vi "Transmitter_type.vi"(8 "error in (no error)":errorcluster, 10 "Transmitter":string="001", 11 "VISA resource name":refnum<visa-resource-name>) -> (0 "error out":errorcluster, 1 "Vacuum gauge type":string, 2 "Transmitter type":string, 3 "VISA resource name 2":refnum<visa-resource-name>)   [LabVIEW 2010]
panel:
  out "concatenated string":string
  out "octal integer string":string
  out "sum":u8
  out "unsigned byte array":u8[](array[numeric])
  out "*(type *) &x":string
  out "Numeric":u8
  out "read buffer":string
  out "return count":u32
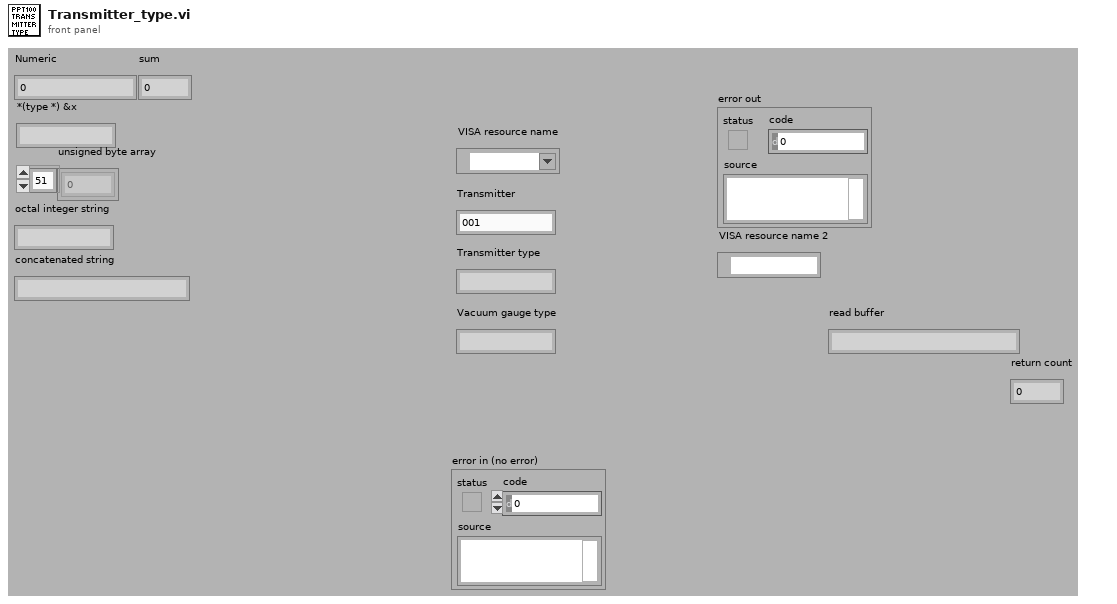
[diagram p1: front panel]
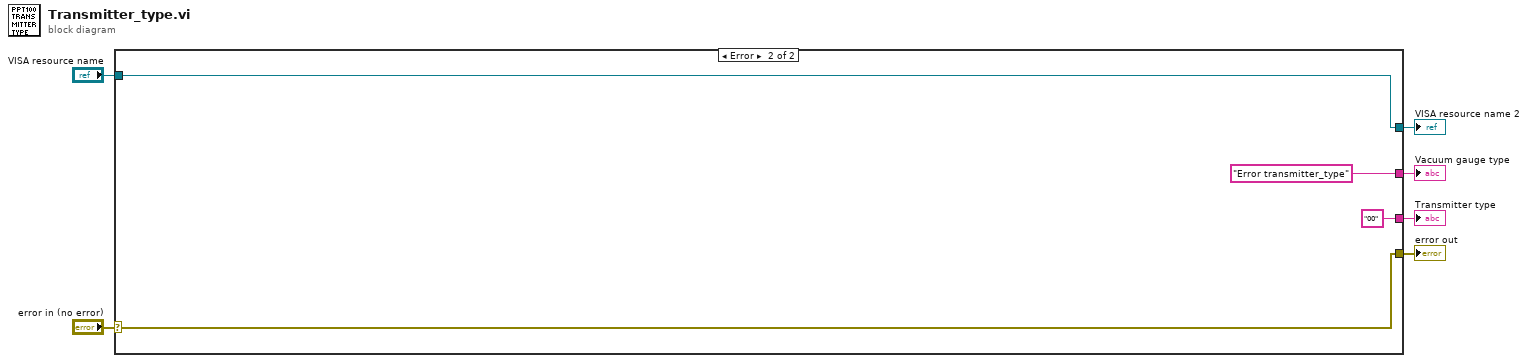
[diagram p0: block diagram]
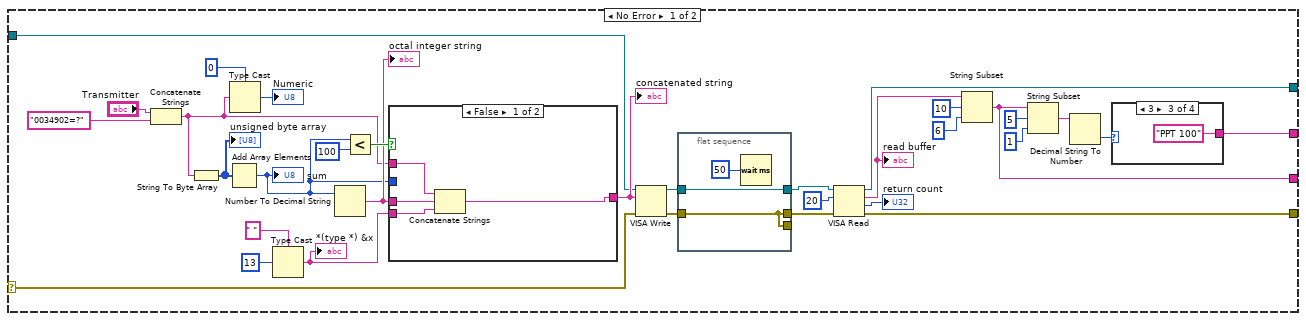
[diagram p2: hidden frame]
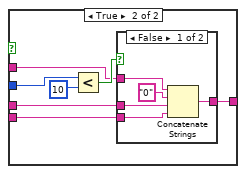
[diagram p3: hidden frame]
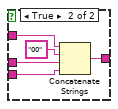
[diagram p4: hidden frame]
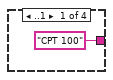
[diagram p5: hidden frame]
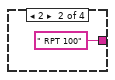
[diagram p6: hidden frame]
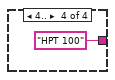
[diagram p7: hidden frame]
diagram:
  n1 = case shown="Error" "error in (no error)" {
    selector: "error in (no error)" -> [w10 w70]
    tunnel: "VISA resource name" -> [w11 w71]
    tunnel: [w37 w70] -> w5
    tunnel: [w36 w71] -> w3
    tunnel: [w28 "00" ("read buffer")] -> w2
    tunnel: [w24 "Error transmitter_type" ("read buffer")] -> w1
    frame No Error {
      n2 = Concatenate Strings("Transmitter", "0034902=?") -> (w9:string)
      n3 = String To Byte Array(string=w9) -> (unsigned byte array=w18:u8[])
      "unsigned byte array" <- w18
      n4 = Add Array Elements(numeric array=w18) -> (sum=w13:u8)
      "sum" <- w13
      n5 = Type Cast(type=u8 0, x=w9) -> (*(type *) &x=→"Numeric":u8)
      n6 = Type Cast(type=" ", x=u8 13 ("Numeric 2")) -> (*(type *) &x=w15:string)
      "*(type *) &x" <- w15
      n7 = Number To Decimal String(number=w13) -> (decimal integer string=w14:string)  [unwired: 1 in]
      "octal integer string" <- w14
      n8 = Less?(x=w13, y=u8 100) -> (x < y?=w16:bool)
      n9 = case shown="False" w16 {
        tunnel: w9 -> [w43 w45]
        tunnel: w15 -> [w41 w47]
        tunnel: w14 -> [w40 w46]
        tunnel: w13 -> [_ w50]
        tunnel: [w42 w44] -> w12
        frame False {
          n10 = Concatenate Strings(w43, w40, w41) -> (w42:string)
        }
        frame True {
          n11 = Less?(x=w50, y=u8 10) -> (x < y?=w48:bool)
          n12 = case shown="False" w48 {
            tunnel: w47 -> [w54 w59]
            tunnel: w46 -> [w53 w58]
            tunnel: w45 -> [w52 w57]
            tunnel: [w51 w56] -> w44
            frame False {
              n13 = Concatenate Strings(w52, "0" ("string"), w53, w54) -> (w51:string)
            }
            frame True {
              n14 = Concatenate Strings(w57, "00" ("string"), w58, w59) -> (w56:string)
            }
          }
        }
      }
      "concatenated string" <- w12
      n15 = VISA Write(VISA resource name=w11, write buffer=w12, error in (no error)=w10) -> (VISA resource name out=w8:refnum<visa-resource-name>, error out=w7:errorcluster)  [unwired: 1 out]
      n16 = flat-sequence {
        tunnel: [w66] -> w33
        tunnel: [w65] -> _
        tunnel: [w65] -> w34
        tunnel: w8 -> [w66]
        tunnel: w7 -> [w65]
        frame #0 {
          n17 = Wait (ms)(milliseconds to wait=u32 50) -> ()  [unwired: 1 out]
        }
      }
      n18 = VISA Read(VISA resource name=w33, byte count=u32 20, error in (no error)=w34) -> (VISA resource name out=w36:refnum<visa-resource-name>, read buffer=w31:string, return count=→"return count":u32, error out=w37:errorcluster)
      "read buffer" <- w31
      n19 = String Subset(string=w31, offset (0)=10, length (rest)=6 ("length (rest)")) -> (substring=w28:string)
      n20 = String Subset(string=w28, offset (0)=5, length (rest)=1 ("length (rest)")) -> (substring=w25:string)
      n21 = Decimal String To Number(string=w25) -> (number=w23:i32)  [unwired: 2 in, 1 out]
      n22 = case shown="3" w23 {
        tunnel: ["CPT 100" ("octal integer string") " RPT 100" ("octal integer string") "PPT 100" ("octal integer string") "HPT 100" ("octal integer string")] -> w24
        frame ..1 {
        }
        frame 2 {
        }
        frame 3 {
        }
        frame 4.. {
        }
      }
    }
    frame Error {
    }
  }
  "error out" <- w5
  "VISA resource name 2" <- w3
  "Transmitter type" <- w2
  "Vacuum gauge type" <- w1
